vi "Set Button State.vi"(8 "error in (no error)":errorcluster, 9 "Button State":T1, 10 "Button Index":i32, 11 "Toolbar Control in":refnum<class "Toolbar Control.lvclass">) -> (0 "error out":errorcluster, 2 "Toolbar Image":picture, 3 "Toolbar Control out":refnum<class "Toolbar Control.lvclass">)   [LabVIEW 2011, in "Toolbar Control.lvclass"]
doc: "This VI sets the buttons specified by their indexes <B>Button Indexe</B> to the states <B>Button State</B>. If <B>Button State</B> is not provided they default to enabled.\n\n-------------\nDeveloped by Brian Hoover (hooovahh)"
uses:
  Toolbar Control.lvclass
  Controls/Button State.ctl
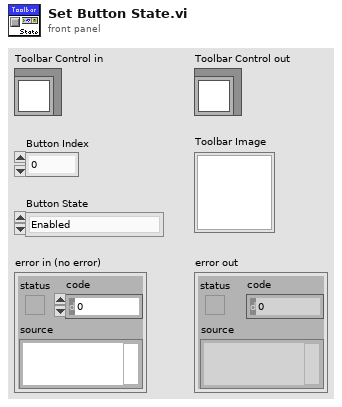
[diagram p1: front panel]
types:
  T1 = typedef "Toolbar Control.lvclass/Button State.ctl" = enum8{"Enabled", "Disabled", "Disabled and Grayed Out"}
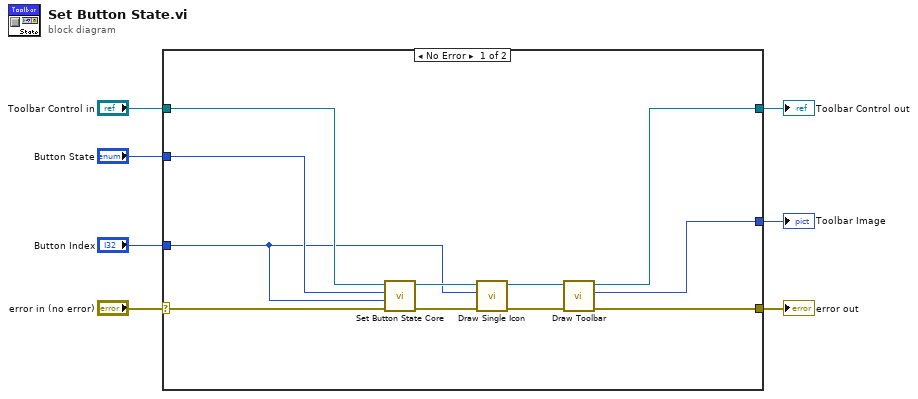
[diagram p0: block diagram]
diagram:
  n1 = case shown="No Error" "error in (no error)" {
    selector: "error in (no error)" -> [w17 w20]
    tunnel: [w15 w20] -> w6
    tunnel: [w14 w19] -> w4
    tunnel: "Toolbar Control in" -> [w18 w19]
    tunnel: "Button State" -> [w16 _]
    tunnel: "Button Index" -> [w9 _]
    tunnel: [w8 _] -> w1
    frame No Error {
      n2 = call "Set Button State Core.vi"("error in (no error)"=w17, "Button Index"=w9, "Button State"=w16, "Toolbar Control in"=w18) -> ("error out"=w13:errorcluster, "Toolbar Control out"=w12:refnum<class "Toolbar Control.lvclass">)  [unwired: 6 in]
      n3 = call "Draw Single Icon.vi"("error in (no error)"=w13, "Icon Index"=w9, "Toolbar Control in"=w12) -> ("error out"=w10:errorcluster, "Toolbar Control out"=w11:refnum<class "Toolbar Control.lvclass">)  [unwired: 7 in]
      n4 = call "Draw Toolbar.vi"("error in (no error)"=w10, "Toolbar Control in"=w11) -> ("error out"=w15:errorcluster, "Toolbar Image"=w8:picture, "Toolbar Control out"=w14:refnum<class "Toolbar Control.lvclass">)  [unwired: 7 in]
    }
    frame Error {
    }
  }
  "error out" <- w6
  "Toolbar Control out" <- w4
  "Toolbar Image" <- w1
